vi "Run Action.vi"(8 "error in (no error)":errorcluster, 10 "Project Builder in":refnum<class "Project Builder.lvclass">, 11 "Project Action":refnum<class "Project Action.lvclass">) -> (0 "error out":errorcluster, 1 "Success?":bool, 3 "Report Array":refnum<class "Report Data.lvclass">[](array[class]))   [LabVIEW 2020]
uses:
  Project Action.lvclass
  Data/Report Data/Report Data.lvclass
  Project Builder/Project Builder.lvclass
  Data/Report Data/Report Data.lvclass/Report Data.ctl
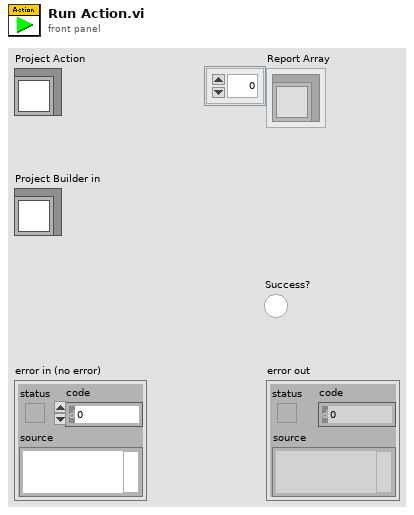
[diagram p1: front panel]
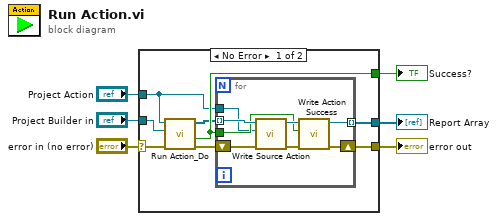
[diagram p0: block diagram]
diagram:
  n1 = case shown="No Error" "error in (no error)" {
    selector: "error in (no error)" -> [w8 w23]
    tunnel: [w10 w23] -> w5
    tunnel: [w12 _] -> w3
    tunnel: "Project Action" -> [w9 _]
    tunnel: [w14 _] -> w2
    tunnel: "Project Builder in" -> [w7 _]
    frame No Error {
      n2 = call-dynamic "Run Action_Do.vi"("error in (no error)"=w8, "Project Builder in"=w7, "Project Action"=w9) -> ("error out"=w11:errorcluster, "Success?"=w14:bool, "Report Array"=w13:refnum<class "Report Data.lvclass">[])  [unwired: 6 in]
      n3 = for {
        tunnel: w13 -> [w22] mode=indexing
        tunnel: w14 -> [w20]
        tunnel: w9 -> [w16]
        tunnel: [w19] -> w12 mode=indexing
        shift-right: [w17] -> w10
        shift-left: w11 -> [w15]
        n4 = call "Write Source Action.vi"("error in (no error)"=w15, "Source Action"=w16, "Report Data in"=w22) -> ("error out"=w18:errorcluster, "Report Data out"=w21:refnum<class "Report Data.lvclass">)  [unwired: 7 in]
        n5 = call "Write Action Success.vi"("error in (no error)"=w18, "Action Success?"=w20, "Report Data in"=w21) -> ("error out"=w17:errorcluster, "Report Data out"=w19:refnum<class "Report Data.lvclass">)  [unwired: 7 in]
      }
    }
    frame Error {
    }
  }
  "error out" <- w5
  "Report Array" <- w3
  "Success?" <- w2
